vi "rscmxpbase_FormatActiveSIMSlotRepCapBoolean_ReadCallback.vi"(5 "Attribute":T1={"Identifier"="", "Descriptive Name"="", "Data Type"=enum."Integer 32", "Command"="", "Access"=enum."Read/Write", "Range Table"="", "Read Callback"="", "Write Callback"="", "Supported Models"="", "Instrument Options"="", "Index"=0, "OPC Wait"=FALSE, "No Status Check"=FALSE, "Cache Only"=FALSE}, 7 "Repeated Capability":string, 8 "error in (no error)":errorcluster, 11 "VISA resource name":refnum<visa-resource-name>) -> (0 "error out":errorcluster, 2 "Attribute Value Boolean":bool, 3 "VISA resource name out":refnum<visa-resource-name>)   [LabVIEW 2015, in "Rohde&Schwarz CMXP Base.lvlib"]
doc: "Replaces <ActiveDUTSIMSlot> with the value of RSCMXPBASE_ATTR_SELECT_ACTIVE_DUT_SIM_SLOT."
uses:
  <instrlib>/Rohde&Schwarz CMXP Base/Rohde&Schwarz CMXP Base.lvlib
  <instrlib>/Rohde&Schwarz CMXP Base/Private/rsidr_core.llb/type_Attribute.ctl
  <instrlib>/Rohde&Schwarz CMXP Base/Private/rsidr_core.llb/type_Attribute_Data_Type.ctl
  <instrlib>/Rohde&Schwarz CMXP Base/Private/rsidr_core.llb/type_ReadWriteAccess.ctl
  <instrlib>/Rohde&Schwarz CMXP Base/Private/rsidr_core.llb/rsidr_core.lvlib
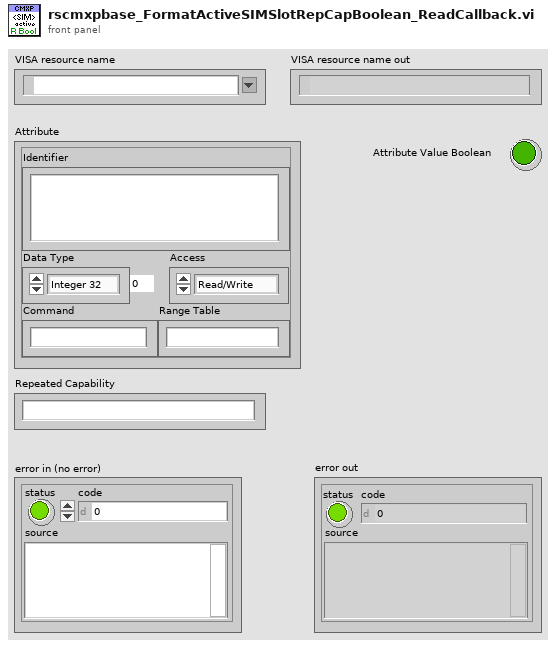
[diagram p1: front panel]
types:
  T1 = typedef "Rohde&Schwarz CMXP Base.lvlib/rsidr_core.lvlib/type_Attribute.ctl" = cluster{"Identifier":string, "Descriptive Name":string, "Data Type":T2, "Command":string, "Access":T3, "Range Table":string, "Read Callback":string, "Write Callback":string, "Supported Models":string, "Instrument Options":string, "Index":i32, "OPC Wait":bool, "No Status Check":bool, "Cache Only":bool}
  T2 = typedef "Rohde&Schwarz CMXP Base.lvlib/rsidr_core.lvlib/type_Attribute_Data_Type.ctl" = enum16{"Integer 32", "Double", "String", "Boolean", "None", "Integer 64", "RawString"}
  T3 = typedef "Rohde&Schwarz CMXP Base.lvlib/rsidr_core.lvlib/type_ReadWriteAccess.ctl" = enum16{"Read Only", "Write Only", "Read/Write"}
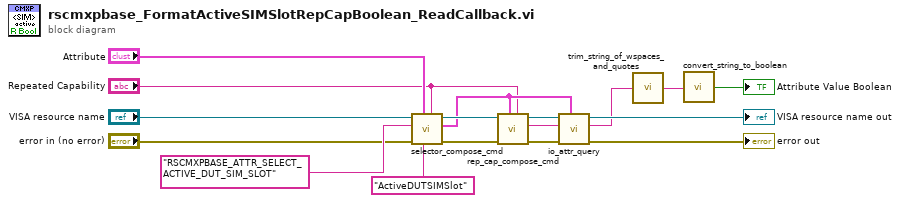
[diagram p0: block diagram]
diagram:
  n1 = call <instrlib>:"selector_compose_cmd.vi"("Repeated Capability"="Repeated Capability", "Selector Name"="ActiveDUTSIMSlot", "Attribute"="Attribute", "error in"="error in (no error)", "Selector Attribute ID"="RSCMXPBASE_ATTR_SELECT_ACTIVE_DUT_SIM_SLOT", "VISA resource name"="VISA resource name") -> ("error out"=w16:errorcluster, "Attribute out"=w11:T1, "VISA resource name out"=w15:refnum<visa-resource-name>)  [unwired: 3 in]
  n2 = call <instrlib>:"rep_cap_compose_cmd.vi"("Repeated Capability"="Repeated Capability", "Attribute"=w11, "error in"=w16, "VISA resource name"=w15) -> ("error out"=w13:errorcluster, "Command out"=w12:string, "VISA resource name out"=w14:refnum<visa-resource-name>)  [unwired: 5 in]
  n3 = call <instrlib>:"io_attr_query.vi"("Attribute"=w11, "error in"=w13, "write buffer"=w12, "VISA resource name"=w14) -> ("error out"=→"error out":errorcluster, "read buffer"=w1:string, "VISA resource name out"=→"VISA resource name out":refnum<visa-resource-name>)  [unwired: 5 in]
  n4 = call <instrlib>:"trim_string_of_wspaces_and_quotes.vi"("String in"=w1) -> ("String out"=w3:string)  [unwired: 4 in]
  n5 = call <instrlib>:"convert_string_to_boolean.vi"("String in"=w3) -> ("boolean value out"=→"Attribute Value Boolean":bool)  [unwired: 4 in]
